vi "Main Rachel.vi"() -> ()   [LabVIEW 2017]
uses:
  Calibrated Oculus Data.ctl
panel:
  out "2D Picture":picture
  in  "Hold":bool
  out "error out":errorcluster
  out "Raw Oculus Data":T1
  out "Calibrated Oculus Data":T2
  in  "error in":errorcluster
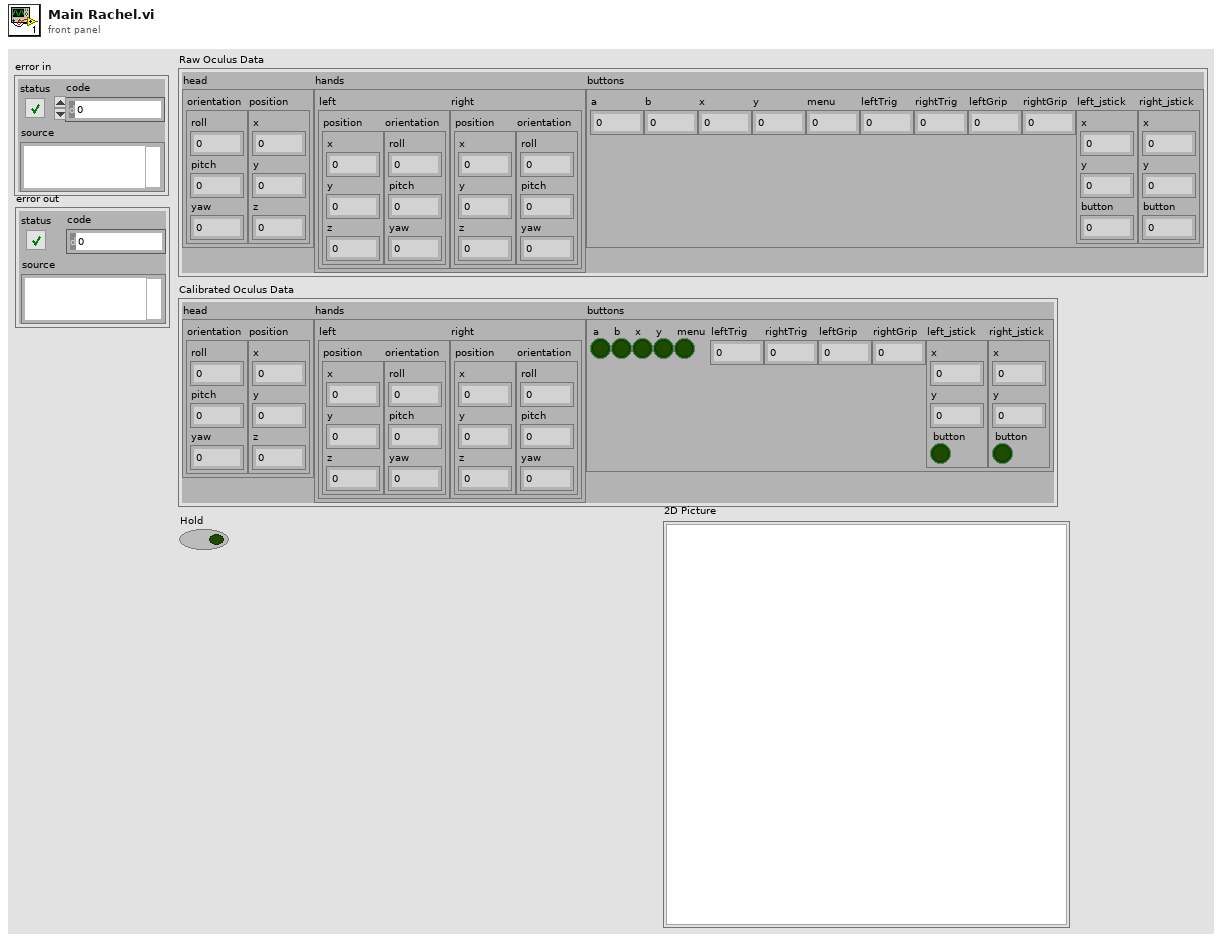
[diagram p1: front panel]
types:
  T1 = cluster{"head":cluster{"orientation":cluster{"roll":dbl, "pitch":dbl, "yaw":dbl}, "position":cluster{"x":dbl, "y":dbl, "z":dbl}}, "hands":cluster{"left":cluster{"position":cluster{"x":dbl, "y":dbl, "z":dbl}, "orientation":cluster{"roll":dbl, "pitch":dbl, "yaw":dbl}}, "right":cluster{"position":cluster{"x":dbl, "y":dbl, "z":dbl}, "orientation":cluster{"roll":dbl, "pitch":dbl, "yaw":dbl}}}, "buttons":cluster{"a":i32, "b":i32, "x":i32, "y":i32, "menu":i32, "leftTrig":dbl, "rightTrig":dbl, "leftGrip":dbl, "rightGrip":dbl, "left_jstick":cluster{"x":dbl, "y":dbl, "button":i32}, "right_jstick":cluster{"x":dbl, "y":dbl, "button":i32}}}
  T2 = typedef "Calibrated Oculus Data.ctl" = cluster{"head":cluster{"orientation":cluster{"roll":dbl, "pitch":dbl, "yaw":dbl}, "position":cluster{"x":dbl, "y":dbl, "z":dbl}}, "hands":cluster{"left":cluster{"position":cluster{"x":dbl, "y":dbl, "z":dbl}, "orientation":cluster{"roll":dbl, "pitch":dbl, "yaw":dbl}}, "right":cluster{"position":cluster{"x":dbl, "y":dbl, "z":dbl}, "orientation":cluster{"roll":dbl, "pitch":dbl, "yaw":dbl}}}, "buttons":cluster{"a":bool, "b":bool, "x":bool, "y":bool, "menu":bool, "leftTrig":dbl, "rightTrig":dbl, "leftGrip":dbl, "rightGrip":dbl, "left_jstick":cluster{"x":dbl, "y":dbl, "button":bool}, "right_jstick":cluster{"x":dbl, "y":dbl, "button":bool}}}
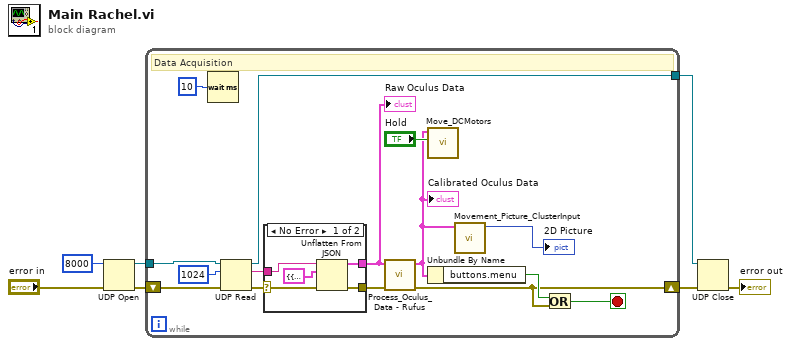
[diagram p0: block diagram]
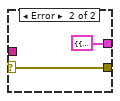
[diagram p2: hidden frame]
diagram:
  n1 = UDP Open(8:"error in", 11:8000) -> (port=w2:refnum<k16>, 0:w1:errorcluster)  [unwired: 3 in, 1 out]
  n2 = while "Data Aquisition" {
    shift-right: [w13] -> w5
    shift-left: w1 -> [w20]
    tunnel: [w19] -> w4
    tunnel: w2 -> [w11]
    stop <- w12 stop-if-true
    # "Data Acquisition"
    n3 = Wait (ms)(milliseconds to wait=u32 10) -> ()  [unwired: 1 out]
    n4 = UDP Read(connection ID=w11, max size (548)=1024, 8:w20) -> (data out=w21:string, error out=w22:errorcluster, 3:w19:refnum<k16>)  [unwired: 1 in, 2 out]
    n5 = case shown="No Error" w22 {
      selector: w22 -> [w27 w29]
      tunnel: [w26 w29] -> w14
      tunnel: w21 -> [w25 _]
      tunnel: [w24 T1 {"head"={"orientation"={"roll"=0.0, "pitch"=0.0, "yaw"=0.0}, "position"={"x"=0.0, "y"=0.0, "z"=0.0}}, "hands"={"left"={"position"={"x"=0.0, "y"=0.0, "z"=0.0}, "orientation"={"roll"=0.0, "pitch"=0.0, "yaw"=0.0}}, "right"={"position"={"x"=0.0, "y"=0.0, "z"=0.0}, "orientation"={"roll"=0.0, "pitch"=0.0, "yaw"=0.0}}}, "buttons"={"a"=0, "b"=0, "x"=0, "y"=0, "menu"=0, "leftTrig"=0.0, "rightTrig"=0.0, "leftGrip"=0.0, "rightGrip"=0.0, "left_jstick"={"x"=0.0, "y"=0.0, "button"=0}, "right_jstick"={"x"=0.0, "y"=0.0, "button"=0}}}] -> w16
      frame No Error {
        n6 = Unflatten From JSON(JSON string=w25, type and defaults=T1 {"head"={"orientation"={"roll"=0.0, "pitch"=0.0, "yaw"=0.0}, "position"={"x"=0.0, "y"=0.0, "z"=0.0}}, "hands"={"left"={"position"={"x"=0.0, "y"=0.0, "z"=0.0}, "orientation"={"roll"=0.0, "pitch"=0.0, "yaw"=0.0}}, "right"={"position"={"x"=0.0, "y"=0.0, "z"=0.0}, "orientation"={"roll"=0.0, "pitch"=0.0, "yaw"=0.0}}}, "buttons"={"a"=0, "b"=0, "x"=0, "y"=0, "menu"=0, "leftTrig"=0.0, "rightTrig"=0.0, "leftGrip"=0.0, "rightGrip"=0.0, "left_jstick"={"x"=0.0, "y"=0.0, "button"=0}, "right_jstick"={"x"=0.0, "y"=0.0, "button"=0}}}, error in (no error)=w27) -> (value=w24:T1, error out=w26:errorcluster)  [unwired: 4 in]
      }
      frame Error {
      }
    }
    "Raw Oculus Data" <- w16
    n7 = call "Process_Oculus_Data - Rufus.vi"("error in"=w14, "Raw Oculus Data"=w16) -> ("error out"=w13:errorcluster, "Calibrated Oculus Data"=w9:T2)  [unwired: 7 in, 1 out]
    "Calibrated Oculus Data" <- w9
    n8 = call "Move_DCMotors.vi"("Hold"="Hold", "Oculus Data"=w9) -> ()  [unwired: 10 in]
    n9 = Unbundle By Name(w9) -> ("buttons.menu"=w15:bool)
    n10 = call "Movement_Picture_ClusterInput.vi"("Oculus Data out"=w9) -> ("2D Picture"=→"2D Picture":picture)  [unwired: 10 in]
    n11 = Or(x=w15, y=w13) -> (x .or. y?=w12:bool)
  }
  n12 = UDP Close(connection ID=w4, 8:w5) -> (error out=→"error out":errorcluster)  [unwired: 1 out]
